vi "garage.vi"() -> ()   [LabVIEW 2014]
uses:
  <vilib>/vision/driver/NI_Vision_Acquisition_Software.lvlib
  <vilib>/vision/Image Controls.llb/IMAQ Image.ctl
panel:
  out "Array":T1(array[cluster])
  out "calibration time":u32
  in  "stop":bool
  out "Image Out":T2
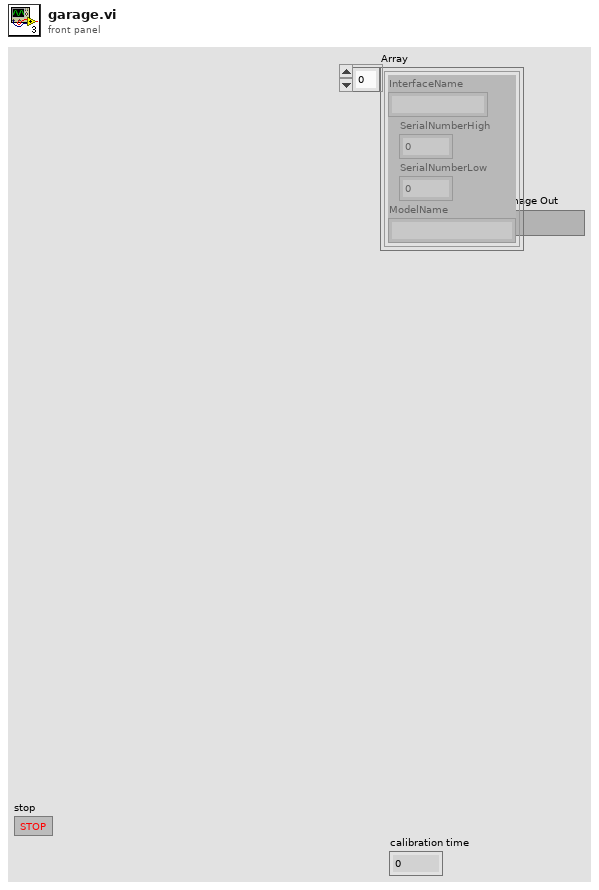
[diagram p1: front panel]
types:
  T1 = cluster{"InterfaceName":string, "SerialNumberHigh":u32, "SerialNumberLow":u32, "ModelName":string}[]
  T2 = typedef "IMAQ Image.ctl" = refnum<image>
  T3 = typedef "IMAQdx.ctl" = refnum<k21>
  T4 = cluster{"Type":u32, "Version":u32, "Flags":u32, "SerialNumberHigh":u32, "SerialNumberLow":u32, "BusType":u32, "InterfaceName":string, "VendorName":string, "ModelName":string, "CameraFileName":string, "CameraAttributeURL":string}[]
  T5 = cluster{"InterfaceName":string, "SerialNumberHigh":u32, "SerialNumberLow":u32, "ModelName":string}
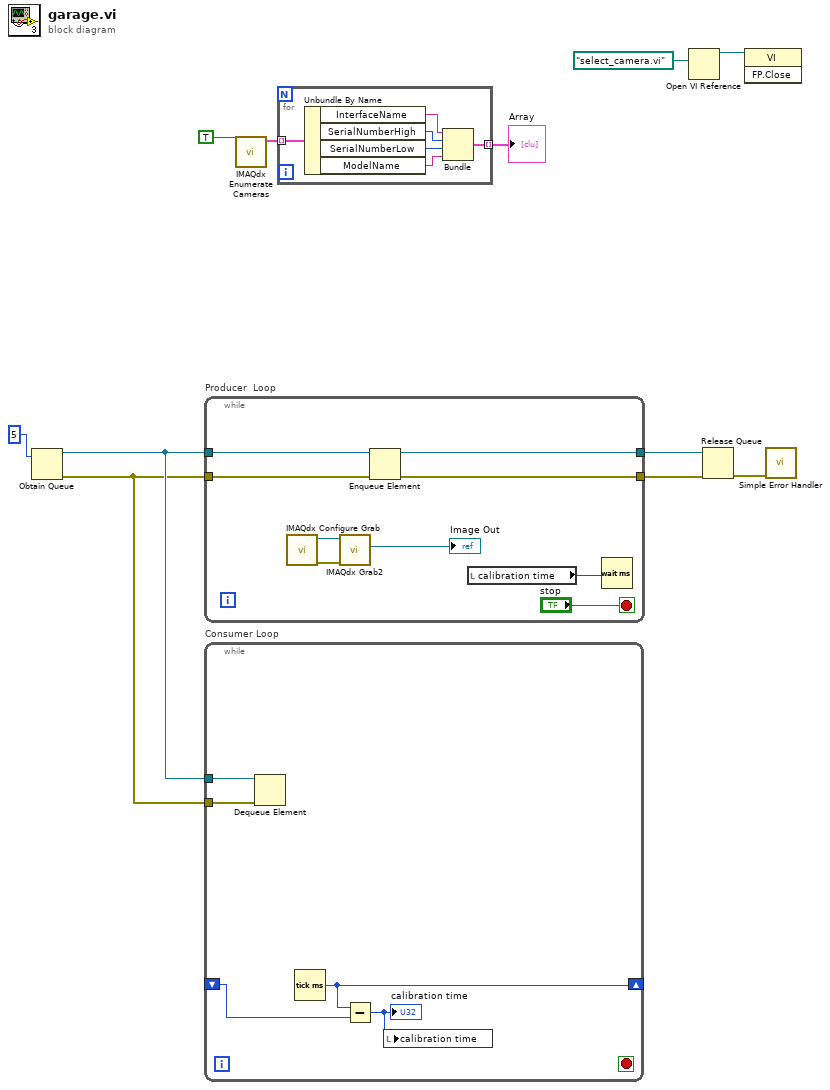
[diagram p0: block diagram]
diagram:
  n1 = Obtain Queue(max queue size (-1, unlimited)=5) -> (queue out=w10:refnum<queue>, error out=w9:errorcluster)  [unwired: 4 in, 1 out]
  n2 = while "Producer  Loop" {
    tunnel: w10 -> [w19]
    tunnel: w9 -> [w16]
    tunnel: [w18] -> w8
    tunnel: [w17] -> w7
    stop <- "stop" stop-if-true
    # "Pro"
    n3 = call <vilib>:"IMAQdx Configure Grab.vi"() -> ("error out"=w12:errorcluster, "Session Out"=w13:T3)  [unwired: 10 in]
    n4 = call <vilib>:"IMAQdx Grab2.vi"("error in"=w12, "Session In"=w13) -> ("Image Out"=→"Image Out":T2)  [unwired: 6 in, 3 out]
    n5 = Enqueue Element(queue=w19, error in (no error)=w16) -> (queue out=w18:refnum<queue>, error out=w17:errorcluster)  [unwired: 2 in, 1 out]
    n6 = local read "calibration time"() -> (w15:u32)
    n7 = Wait (ms)(milliseconds to wait=w15) -> ()  [unwired: 1 out]
  }
  n8 = while "Consumer Loop" {
    tunnel: w10 -> [w25]
    tunnel: w9 -> [w24]
    shift-right: [w22] -> _
    shift-left: _ -> [w23]
    stop <- _ stop-if-true
    n9 = Dequeue Element(queue=w25, error in (no error)=w24) -> ()  [unwired: 1 in, 4 out]
    n10 = Tick Count (ms)() -> (millisecond timer value=w22:u32)
    n11 = Subtract(x=w22, y=w23) -> (x-y=w21:u32)
    "calibration time" <- w21
    n12 = local write "calibration time"(w21) -> ()
  }
  n13 = call <vilib>:"IMAQdx Enumerate Cameras.vi"("Connected Only? (Yes)"=TRUE) -> ("Camera Information Array"=w5:T4)  [unwired: 9 in, 1 out]
  n14 = for {
    tunnel: w5 -> [w31] mode=indexing
    tunnel: [w28] -> w4 mode=indexing
    n15 = Unbundle By Name(w31) -> ("InterfaceName"=w26:string, "SerialNumberHigh"=w30:u32, "SerialNumberLow"=w29:u32, "ModelName"=w27:string)
    n16 = Bundle("InterfaceName"=w26, "SerialNumberHigh"=w30, "SerialNumberLow"=w29, "ModelName"=w27) -> (w28:T5)  [unwired: 1 in]
  }
  "Array" <- w4
  n17 = Open VI Reference(vi path=path "select_camera.vi") -> (vi reference=w1:refnum<vi>)  [unwired: 5 in, 1 out]
  n18 = Release Queue(queue=w8, error in (no error)=w7) -> (error out=w6:errorcluster)  [unwired: 1 in, 2 out]
  n19 = invoke class="VI" method="FP.Close"(reference=w1) -> ()  [unwired: 2 in, 3 out]
  n20 = call <vilib>:"Simple Error Handler.vi"("error in (no error)"=w6) -> ()  [unwired: 4 in, 5 out]
